vi "Teleop_Acquire_Decide.vi"(8 "error in (no error)":errorcluster) -> (0 "error out":errorcluster)   [LabVIEW 2019]
uses:
  <vilib>/Rock Robotics/WPI/Joystick/XBox Buttons Indexer.ctl
  <vilib>/Rock Robotics/WPI/Joystick/XBox Axes Indexer.ctl
  <vilib>/Rock Robotics/WPI/ThirdParty/JAS_Junk/TrajLib/VI/DigSeqLogic_Edge_On.vi
  <vilib>/Rock Robotics/WPI/ThirdParty/JAS_Junk/TrajLib/VI/BoolCmd_Send_Internal.vi
  <vilib>/Rock Robotics/WPI/ThirdParty/JAS_Junk/TrajLib/Rotation2d_CreateAngleDegrees.vi
  <vilib>/Rock Robotics/WPI/ThirdParty/JAS_Junk/TrajLib/VI/BoolCmd_ObtainQueue.vi
  <vilib>/Rock Robotics/WPI/ThirdParty/JAS_Junk/TrajLib/Conv_Deg_Radians.vi
  <vilib>/Rock Robotics/WPI/ThirdParty/JAS_Junk/TrajLib/Rotation2d_CreateAngle.vi
  <vilib>/Rock Robotics/WPI/Utilities/WPI_GetSetVariantRefNum.vi
  <vilib>/Rock Robotics/WPI/Joystick/WPI_JoystickArcadeMapping.vi
  Diff_Drive_System/Diff_Drive_System_Globals.vi
  <vilib>/Rock Robotics/WPI/ThirdParty/JAS_Junk/TrajLib/Trajectory_Library.lvlib
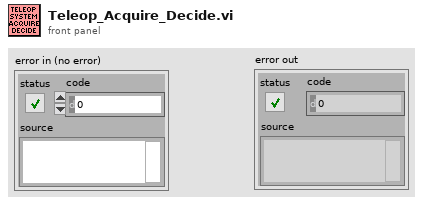
[diagram p1: front panel]
types:
  T1 = typedef "XBox Axes Indexer.ctl" = enum16{"Left X", "Left Y", "Left Trigger", "Right Trigger", "Right X", "Right Y"}
  T2 = typedef "XBox Buttons Indexer.ctl" = enum16{"A", "B", "X", "Y", "Left Bumper", "Right Bumper", "Back", "Start", "Left Joystick", "Right Joystick"}
  T3 = typedef "WPI_JoystickDevRef.ctl" = cluster{"Device":T4}
  T4 = typedef "WPI_JoystickDeviceEnum.ctl" = enum16{"USB 0", "USB 1", "USB 2", "USB 3", "USB 4", "USB 5"}
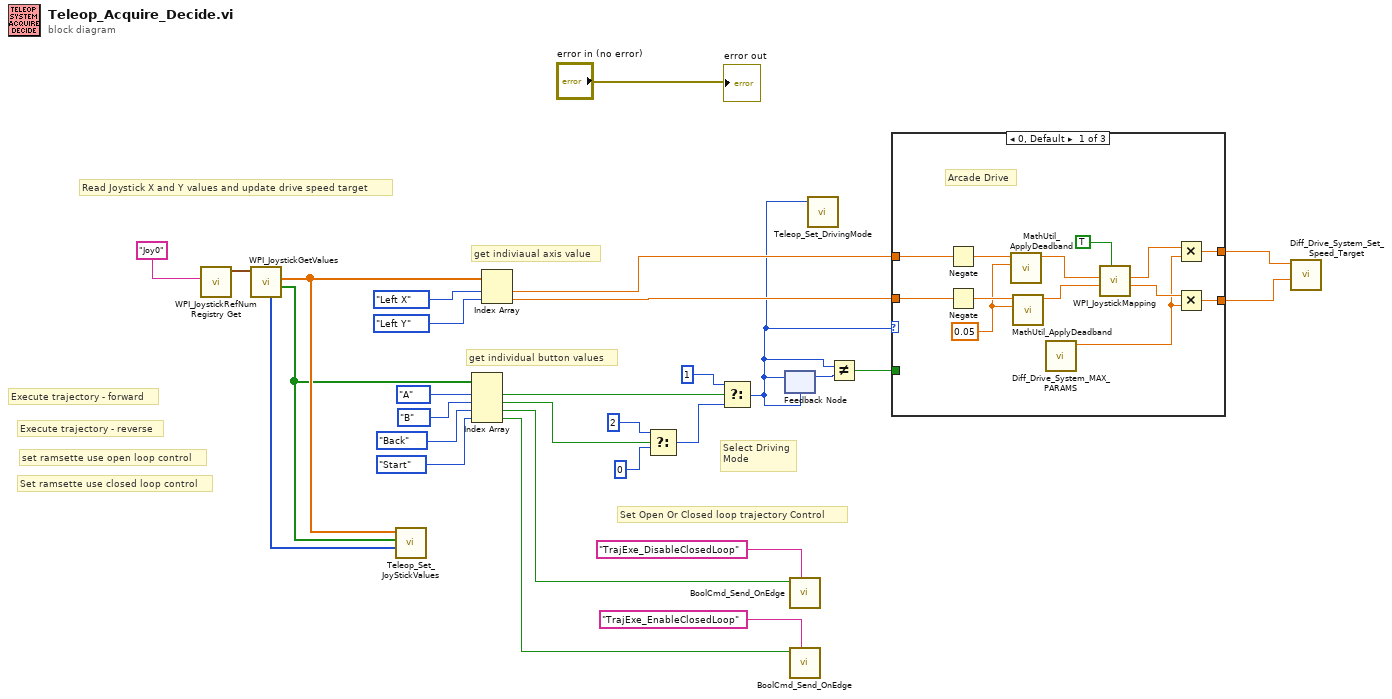
[diagram p0: block diagram]
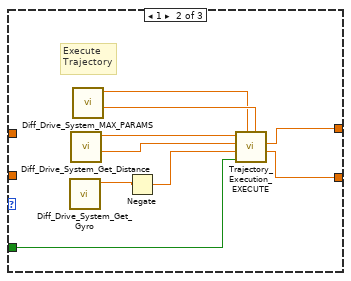
[diagram p2: hidden frame]
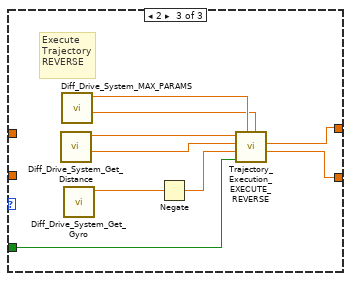
[diagram p3: hidden frame]
diagram:
  # "set ramsette use open loop control"
  # "Set ramsette use closed loop control"
  # "Execute trajectory - reverse"
  # "Execute trajectory - forward"
  # "Set Open Or Closed loop trajectory Control"
  # "Select Driving\nMode"
  # "get individual button values"
  # "get indiviaual axis value"
  # "Read Joystick X and Y values and update drive speed target"
  n1 = call <vilib>:"WPI_JoystickRefNum Registry Get.vi"("refnum name"="Joy0") -> ("JoystickDevRef"=w19:T3)  [unwired: 1 in, 9 out]
  n2 = call <vilib>:"WPI_JoystickGetValues.vi"("JoystickDevRef"=w19) -> ("Buttons"=w3:bool[], "Axes"=w4:dbl[], "POVs"=w2:i16[])  [unwired: 6 in, 2 out]
  n3 = call "Teleop_Set_JoyStickValues.vi"("Joy0-POV"=w2, "Joy0-Buttons"=w3, "Joy0-Axes"=w4) -> ()  [unwired: 9 in]
  n4 = Index Array(array=w3, index #1=XBox_Buttons_Indexer."A" ("XBox Buttons"), index #2=XBox_Buttons_Indexer."B" ("XBox Buttons"), index #3=XBox_Buttons_Indexer."Back" ("XBox Buttons"), index #4=XBox_Buttons_Indexer."Start" ("XBox Buttons")) -> (element #1=w23:bool, element #2=w29:bool, element #3=w10:bool, element #4=w9:bool)
  n5 = Index Array(array=w4, index #1=XBox_Axes_Indexer."Left X" ("XBox Axes"), index #2=XBox_Axes_Indexer."Left Y" ("XBox Axes")) -> (element #1=w20:dbl, element #2=w21:dbl)
  n6 = Select(t=2, s=w29, f=0) -> (s? t:f=w28:i32)
  n7 = Select(t=1, s=w23, f=w28) -> (s? t:f=w1:i32)
  n8 = feedback #1(w1) -> (w24:i32)
  n9 = feedback-in #1(w1) -> ()
  n10 = call <vilib>:"BoolCmd_Send_OnEdge.vi"("Command Name"="TrajExe_DisableClosedLoop", "Value"=w10) -> ()  [unwired: 9 in, 1 out]
  n11 = call <vilib>:"BoolCmd_Send_OnEdge.vi"("Command Name"="TrajExe_EnableClosedLoop", "Value"=w9) -> ()  [unwired: 9 in, 1 out]
  n12 = call "Teleop_Set_DrivingMode.vi"("DrivingMode"=w1) -> ()  [unwired: 11 in]
  n13 = Not Equal?(x=w1, y=w24) -> (x != y?=w25:bool)
  n14 = case shown="0, Default" w1 {
    tunnel: w20 -> [w41 _ _]
    tunnel: w21 -> [w40 _ _]
    tunnel: [w39 w44 w58] -> w16
    tunnel: [w38 w43 w57] -> w15
    tunnel: w25 -> [_ w51 w60]
    frame 0, Default {
      w31 = 0.05 ("Deadband")
      # "Arcade Drive"
      n15 = Negate(x=w41) -> (-x=w34:dbl)
      n16 = Negate(x=w40) -> (-x=w33:dbl)
      n17 = call <vilib>:"MathUtil_ApplyDeadband.vi"("Deadband"=w31, "Value"=w34) -> ("Result"=w35:dbl)  [unwired: 9 in]
      n18 = call <vilib>:"MathUtil_ApplyDeadband.vi"("Deadband"=w31, "Value"=w33) -> ("Result"=w32:dbl)  [unwired: 9 in]
      n19 = call "Diff_Drive_System_MAX_PARAMS.vi"() -> ("Max Speed Ft/Sec"=w30:dbl)  [unwired: 10 in, 1 out]
      n20 = call-poly <vilib>:"WPI_JoystickMapping.vi"("Square Inputs"=TRUE, "Y axis value"=w32, "X axis value"=w35) -> ("Right Motor Value"=w36:dbl, "Left Motor Value"=w37:dbl)  [unwired: 7 in]
      n21 = Multiply(x=w37, y=w30) -> (x*y=w39:dbl)
      n22 = Multiply(x=w36, y=w30) -> (x*y=w38:dbl)
    }
    frame 1 {
      # "Execute\nTrajectory"
      n23 = call "Diff_Drive_System_Get_Gyro.vi"() -> ("Gyro_DEG"=w49:dbl)  [unwired: 10 in, 1 out]
      n24 = call "Diff_Drive_System_Get_Distance.vi"() -> ("Right Distance FT"=w47:dbl, "Left Distance FT"=w48:dbl)  [unwired: 10 in]
      n25 = call "Diff_Drive_System_MAX_PARAMS.vi"() -> ("Effective TrackWidth Ft"=w46:dbl, "Max Speed Ft/Sec"=w45:dbl)  [unwired: 10 in]
      n26 = Negate(x=w49) -> (-x=w50:dbl)
      n27 = call "Trajectory_Execution_EXECUTE.vi"("Track Width FT"=w46, "Max Speed\nFT/SEC"=w45, "Init"=w51, "Gyro Continous\n (inc counterclockwise)"=w50, "Right Distance"=w47, "Left Distance"=w48) -> ("Right Speed Target"=w43:dbl, "Left Speed Target"=w44:dbl)  [unwired: 1 in, 3 out]
    }
    frame 2 {
      # "Execute\nTrajectory\nREVERSE"
      n28 = call "Diff_Drive_System_Get_Distance.vi"() -> ("Right Distance FT"=w54:dbl, "Left Distance FT"=w55:dbl)  [unwired: 10 in]
      n29 = call "Diff_Drive_System_MAX_PARAMS.vi"() -> ("Effective TrackWidth Ft"=w52:dbl, "Max Speed Ft/Sec"=w53:dbl)  [unwired: 10 in]
      n30 = call "Diff_Drive_System_Get_Gyro.vi"() -> ("Gyro_DEG"=w56:dbl)  [unwired: 10 in, 1 out]
      n31 = Negate(x=w56) -> (-x=w59:dbl)
      n32 = call "Trajectory_Execution_EXECUTE_REVERSE.vi"("Track Width FT"=w52, "Max Speed\nFT/SEC"=w53, "Init"=w60, "Gyro Continous\n (inc counterclockwise)"=w59, "Right Distance"=w54, "Left Distance"=w55) -> ("Right Speed Target"=w57:dbl, "Left Speed Target"=w58:dbl)  [unwired: 1 in, 3 out]
    }
  }
  n33 = call "Diff_Drive_System_Set_Speed_Target.vi"("Right Speed Target FT/S"=w15, "Left Speed Target FT/S"=w16) -> ()  [unwired: 10 in]
  "error out" <- "error in (no error)"
